vi "Centrifuge Status.vi"(8 "error in (no error)":errorcluster, 11 "?":T1={"State"=enum."Idle", "Start Time"=timestamp(0 s since 1904-01-01), "Configuration"={"Cycle Period"=0.0, "Manual Entry"=0.0, "Output Device"=enum."Default", "EPOS4 Settings"={"VISA resource name"="", "axis"={"keyHandle"=1, "nodeId"=1}, "Simulated?"=FALSE}}, "Current Time"=timestamp(0 s since 1904-01-01), "First Iteration"=FALSE, "Data"={"Centrifuge Speed"=0.0}, "Process Name"="", "Centrifuge On?"=enum."Off", "Output Error"=FALSE, "Log Started"=FALSE}) -> (0 "error out":errorcluster, 3 "State out":T1={"State"=enum."Idle", "Start Time"=timestamp(0 s since 1904-01-01), "Configuration"={"Cycle Period"=0.0, "Manual Entry"=0.0, "Output Device"=enum."Default", "EPOS4 Settings"={"VISA resource name"="", "axis"={"keyHandle"=1, "nodeId"=1}, "Simulated?"=FALSE}}, "Current Time"=timestamp(0 s since 1904-01-01), "First Iteration"=FALSE, "Data"={"Centrifuge Speed"=0.0}, "Process Name"="", "Centrifuge On?"=enum."Off", "Output Error"=FALSE, "Log Started"=FALSE})   [LabVIEW 2018, in "Centrifuge Module.lvlib" / "Centrifuge Module Engine.lvlib"]
uses:
  Measure Instrument/Centrifuge Module Engine.lvlib
  Measure Instrument/State Cluster.ctl
  Measure Instrument/State Enum.ctl
  Centrifuge Module Settings Cluster.ctl
  EPOS4/Controls/Device Selection.ctl
  EPOS4/Controls/EPOS Communication Settings.ctl
  Tag VIs/Tag FGV Operation Enum.ctl
  Shared Variables/Dynamic Shared Variables.lvlib
  EPOS4/EPOS4.lvlib
  Centrifuge Module.lvlib
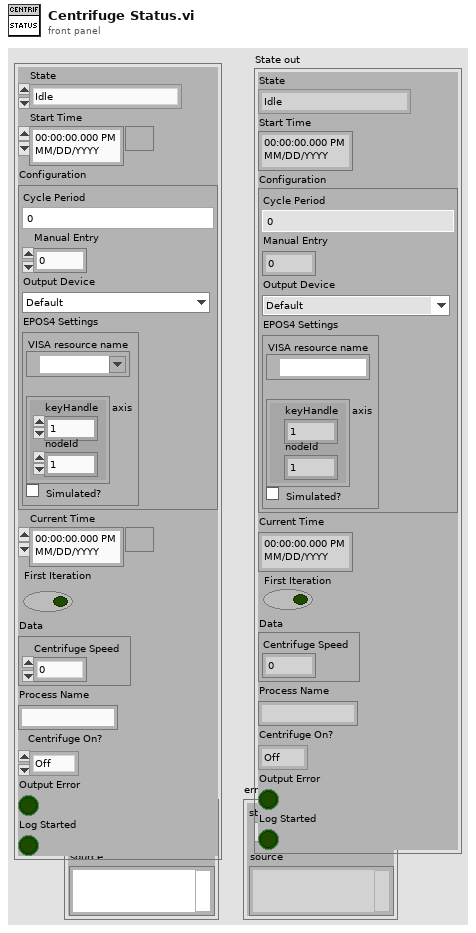
[diagram p1: front panel]
types:
  T1 = typedef "Centrifuge Module.lvlib/Centrifuge Module Engine.lvlib/State Cluster.ctl" = cluster{"State":T2, "Start Time":timestamp, "Configuration":T3, "Current Time":timestamp, "First Iteration":bool, "Data":cluster{"Centrifuge Speed":dbl}, "Process Name":string, "Centrifuge On?":enum16{"Off", "On", "Not Initialized"}, "Output Error":bool, "Log Started":bool}
  T2 = typedef "Centrifuge Module.lvlib/Centrifuge Module Engine.lvlib/State Enum.ctl" = enum16{"Measuring", "Idle", "Paused"}
  T3 = typedef "Centrifuge Module.lvlib/Centrifuge Module Settings Cluster.ctl" = cluster{"Cycle Period":dbl, "Manual Entry":dbl, "Output Device":T4, "EPOS4 Settings":T5}
  T4 = typedef "Device Selection.ctl" = enum16{"Default", "EPOS4"}
  T5 = typedef "EPOS4.lvlib/EPOS Communication Settings.ctl" = cluster{"VISA resource name":refnum<visa-resource-name>, "axis":cluster{"keyHandle":u32, "nodeId":u16}, "Simulated?":bool}
  T6 = typedef "Tag FGV Operation Enum.ctl" = enum16{"Init", "Set Notification Queue", "Create Tag", "Commit", "Write Tag (Numeric)", "Write Tag (Boolean)", "Read All Tags", "Read One Tag", "Delete Tag Category", "Set Alarm Parameters (Numeric)", "Set Alarm Parameters (Boolean)", "Enable All Alarms", "Disable All Alarms", "Delete All Tags", "Read Alarms", "Ack Alarm", "Read Alarm Parameters (Numeric)", "Read Alarm Parameters (Boolean)"}
  T7 = typedef "Centrifuge Module.lvlib/Centrifuge Module Tag Names Cluster.ctl" = cluster{"Centrifuge Speed":string, "Output Device Tag":string}
  T8 = cluster{"positionIs":i32, "velocityIs":i32, "currentIs":i16}
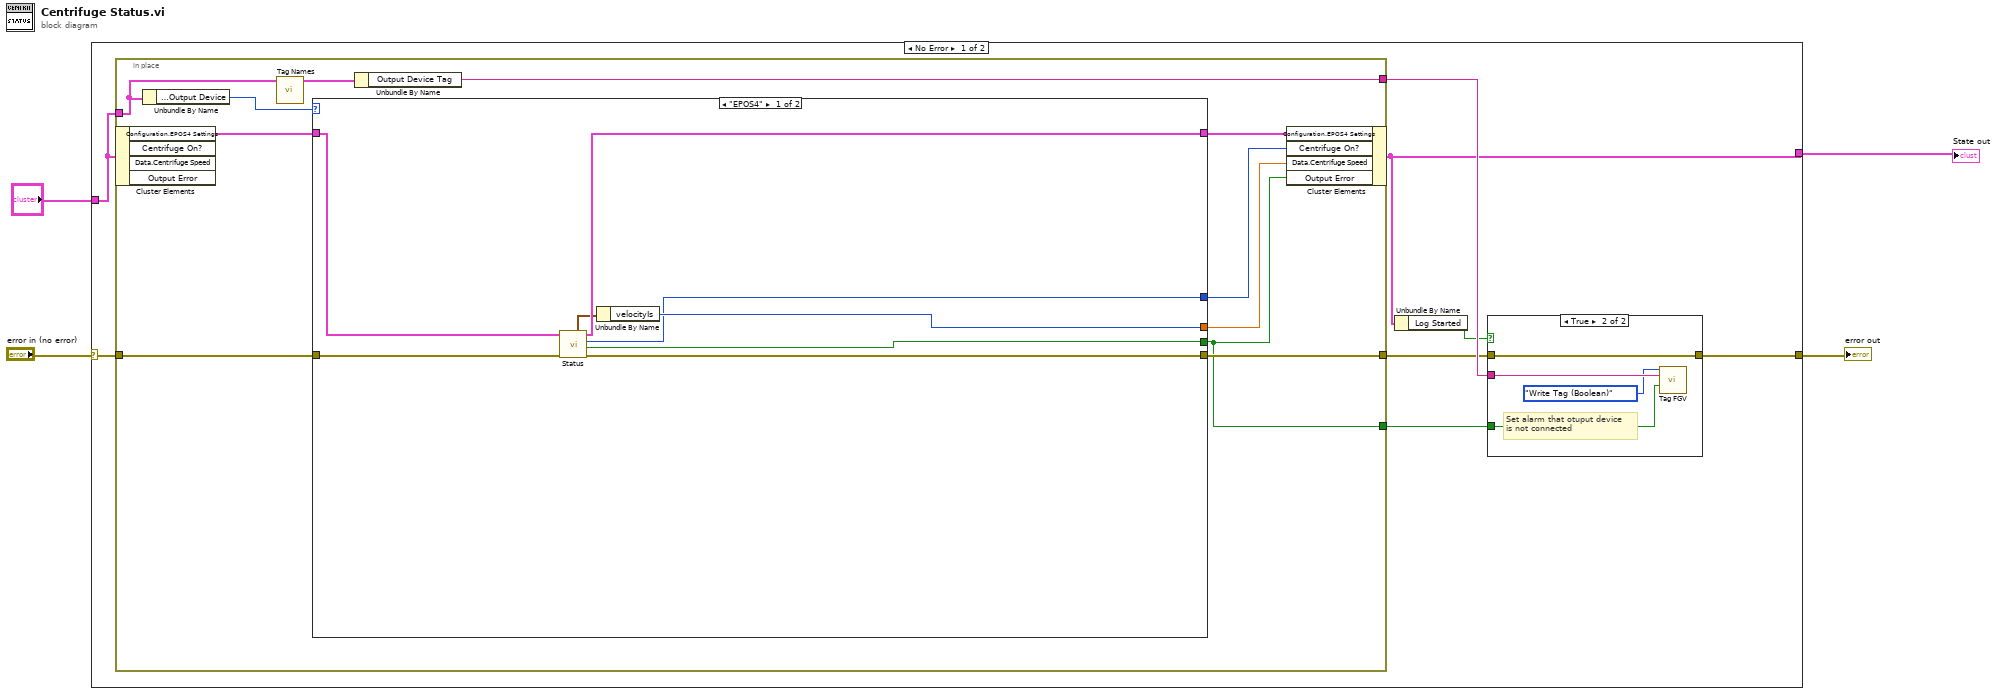
[diagram p0: block diagram]
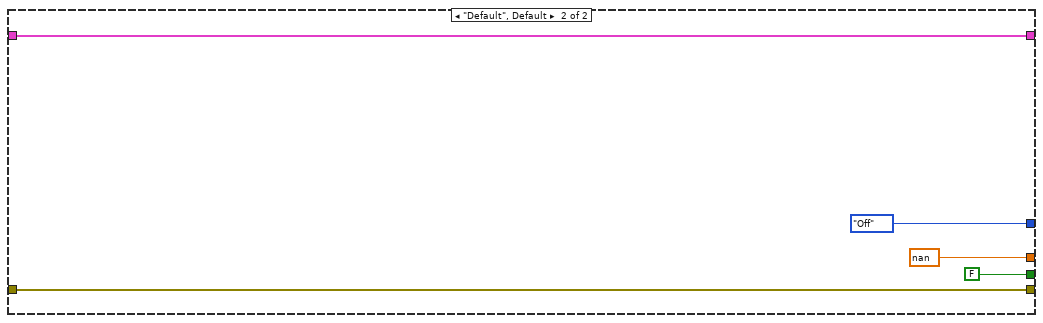
[diagram p2: hidden frame]
diagram:
  n1 = case shown="No Error" "error in (no error)" {
    selector: "error in (no error)" -> [w12 w43]
    tunnel: [w9 w43] -> w3
    tunnel: "?" -> [w6 w42]
    tunnel: [w5 w42] -> w1
    frame No Error {
      n2 = in-place {
        in-place-border: w12 -> [w23]
        in-place-border: [w22] -> w11
        in-place-border: [w21] -> w10
        in-place-border: w6 -> [w18]
        in-place-border: [w15] -> w7
        n3 = in-place-cluster #1(w6) -> ("Configuration.EPOS4 Settings"=w17:T5)  [unwired: 3 out]
        n4 = Unbundle By Name(w18) -> ("Configuration.Output Device"=w19:T4)
        n5 = call "Tag Names.vi"("State In"=w18) -> ("Centrifuge Module Tag Names"=w20:T7)  [unwired: 8 in, 2 out]
        n6 = case "Selected Device" shown="\"EPOS4\"" w19 {
          tunnel: w17 -> [w29 w36]
          tunnel: [w28 w36] -> w16
          tunnel: [w30 w35] -> w21
          tunnel: w23 -> [w31 w35]
          tunnel: [w24 enum16{"Off", "On", "Not Initialized"}."Off" ("Pump On?")] -> w14
          tunnel: [w26 nan ("Flow Rate")] -> w13
          tunnel: [w25 FALSE ("Connection Error")] -> w15
          frame "EPOS4" {
            n7 = call "Status.vi"("error in (no error)"=w31, "EPOS4 Settings In"=w29) -> ("error out"=w30:errorcluster, "Connection Error"=w25:bool, "Centrifuge On?"=w24:enum16{"Off", "On", "Not Initialized"}, "EPOS4 Settings Out"=w28:T5, "axis data"=w27:T8)  [unwired: 5 in]
            n8 = Unbundle By Name(w27) -> ("velocityIs"=w26:i32)
          }
          frame "Default", Default {
          }
        }
        n9 = Unbundle By Name(w20) -> ("Output Device Tag"=w22:string)
        n10 = in-place-cluster #1("Configuration.EPOS4 Settings"=w16, "Centrifuge On?"=w14, "Data.Centrifuge Speed"=w13, "Output Error"=w15) -> (w5:T1)
      }
      n11 = Unbundle By Name(w5) -> ("Log Started"=w8:bool)
      n12 = case shown="True" w8 {
        tunnel: w11 -> [_ w41]
        tunnel: w10 -> [w37 w40]
        tunnel: [w37 w40] -> w9
        tunnel: w7 -> [_ w38]
        frame False {
        }
        frame True {
          # "Set alarm that otuput device\nis not connected"
          n13 = call "Tag FGV.vi"("Operation"=Tag_FGV_Operation_Enum."Write Tag (Boolean)", "Tag Name"=w41, "Data"=w38) -> ()  [unwired: 5 in, 8 out]
        }
      }
    }
    frame Error {
    }
  }
  "error out" <- w3
  "State out" <- w1
